vi "testBench-0#-enumTest.vi"() -> ()   [LabVIEW 2015]
doc: "该模板用于创建生产者／消费者模式的应用程序，以事件驱动的方式，生成队列中的项。如需通过响应事件实现代码的异步执行，同时不影响用户界面的响应速度，可考虑用该模式替代用户界面事件处理器模式。"
panel:
  out "ms":cluster{u32, u32, u32, u32, u32}
  out "算法耗时ms":u32
  out "路径":path
  out "出料信息":enum16{"未检", "废品", "尺寸", "外观", "良品"}(ring)=enum."良品"
  in  "各镜槽向配置修正量":dbl[](array[numeric])=[0.0, 0.0, 0.0, 0.0, 0.0, 0.0, 0.0, 0.0, 0.0, 0.0]
  out "#0判定结果显示":T1={"槽宽最大值"=100.0, "槽宽OK"=FALSE, "铜碎OK"=FALSE, "镀锡OK"=FALSE, "白条OK"=TRUE, "头缺OK"=TRUE, "镜角数值"=0}
  in  "检测控制参数 2":cluster{"槽数":i32, "槽宽上限":dbl, "白条面积上限":dbl}={"槽数"=3, "槽宽上限"=12.0, "白条面积上限"=50.0}
  in  "自动运行":bool
  in  "Quit":bool
  out "完成":bool=TRUE
  in  "文件路径（使用对话框）":path=path "D:/IMGFILES/180404/刀纹/cam5/NG"
  out "Display Image":T2(plugin-control)
  in  "输入簇":errorcluster
  in  "Enqueue Element":bool caption="元素入队列"
  in  "stop":bool caption="停止"
  # "可将错误或警告信息Overlay至图像显示，便于检视"
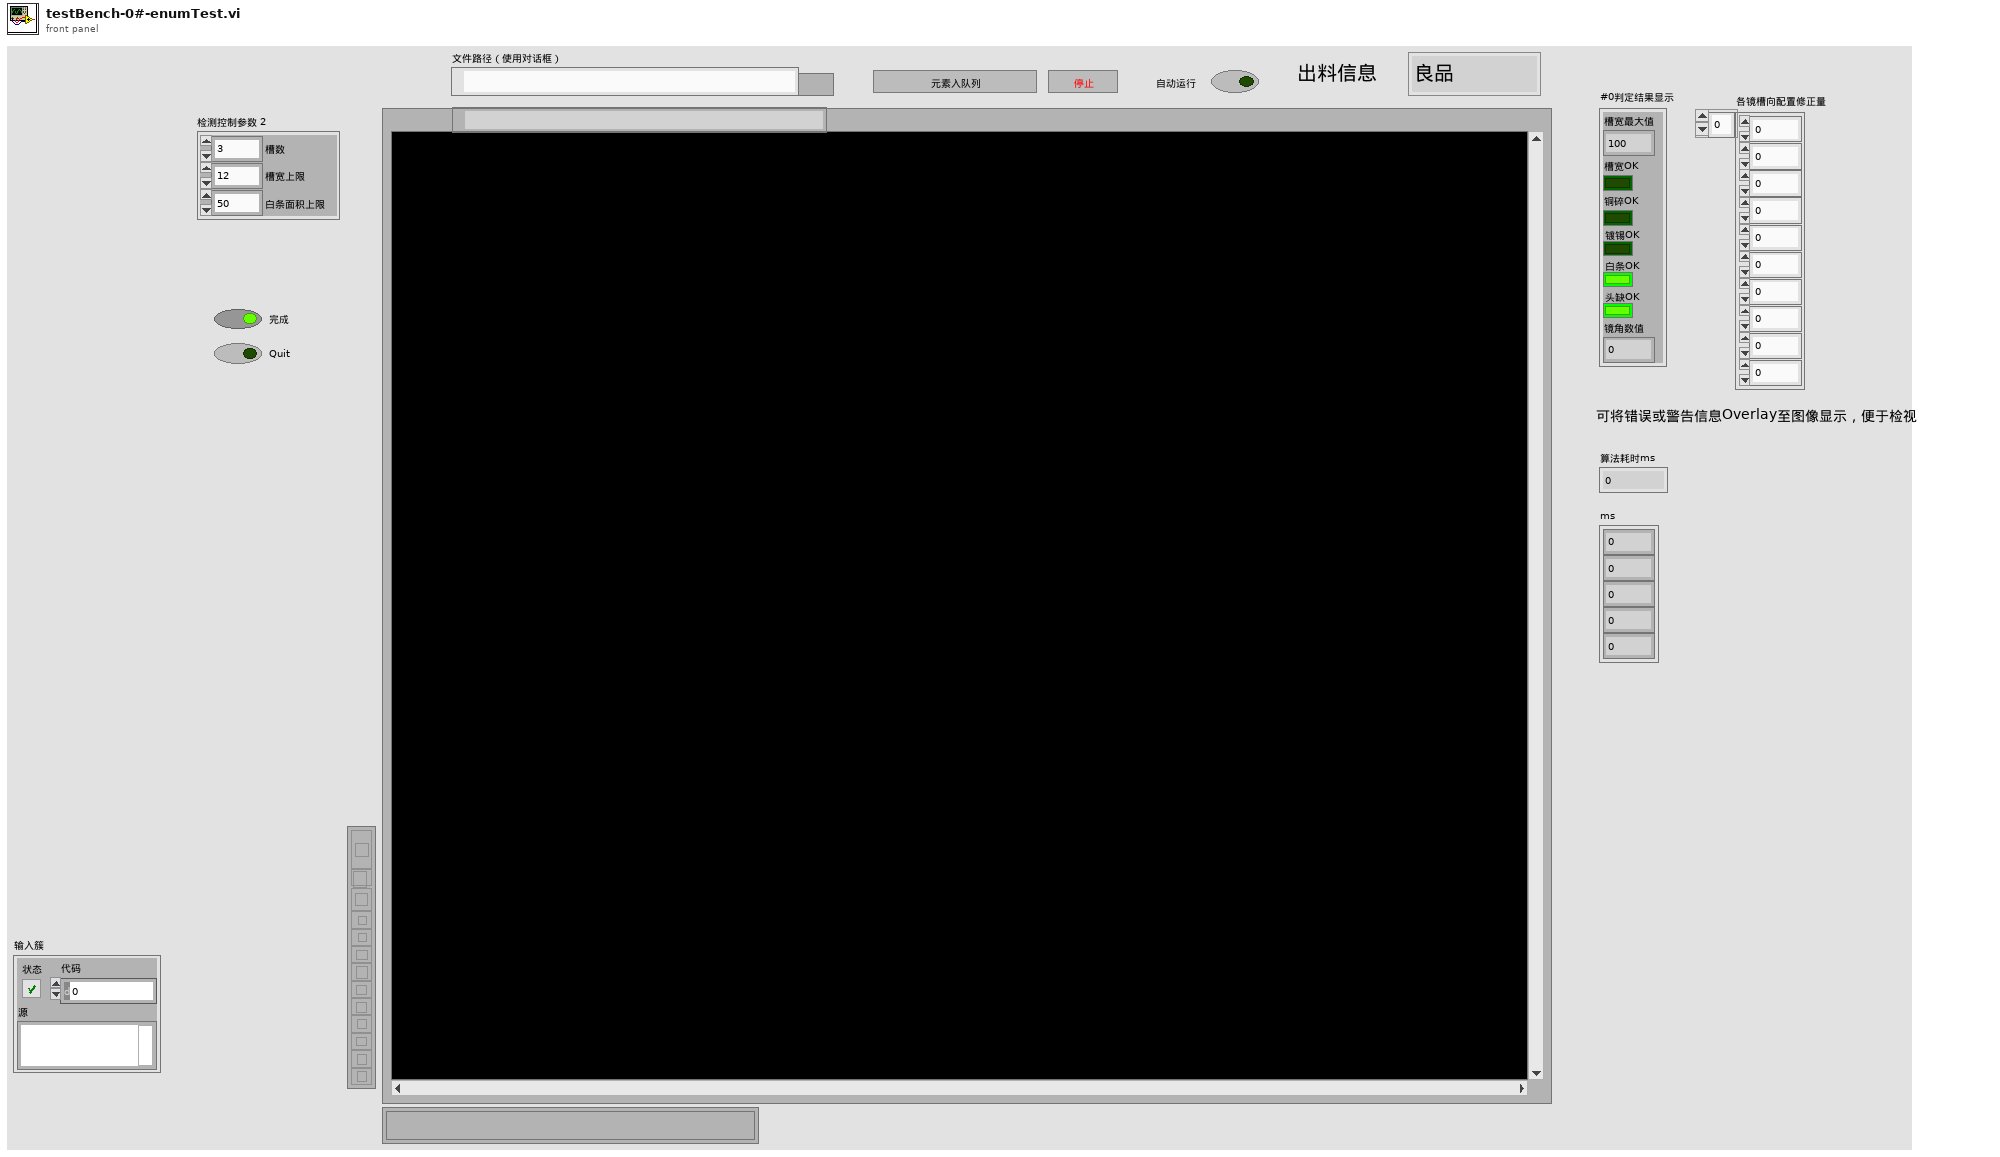
[diagram p1: front panel]
types:
  T1 = cluster{"槽宽最大值":sgl, "槽宽OK":bool, "铜碎OK":bool, "镀锡OK":bool, "白条OK":bool, "头缺OK":bool, "镜角数值":u32}
  T2 = typedef "IMAQ Image.ctl" = refnum<image>
  T3 = typedef "Image Type" = u32
  T4 = cluster{"New Image":T2, "New Image":T2, "New Image":T2, "New Image":T2, "New Image":T2, "New Image":T2, "New Image":T2, "New Image":T2, "New Image":T2, "New Image":T2, "New Image":T2, "New Image":T2, "New Image":T2, "New Image":T2, "New Image":T2, "New Image 2":T2, "New Image 3":T2, "New Image 4":T2}
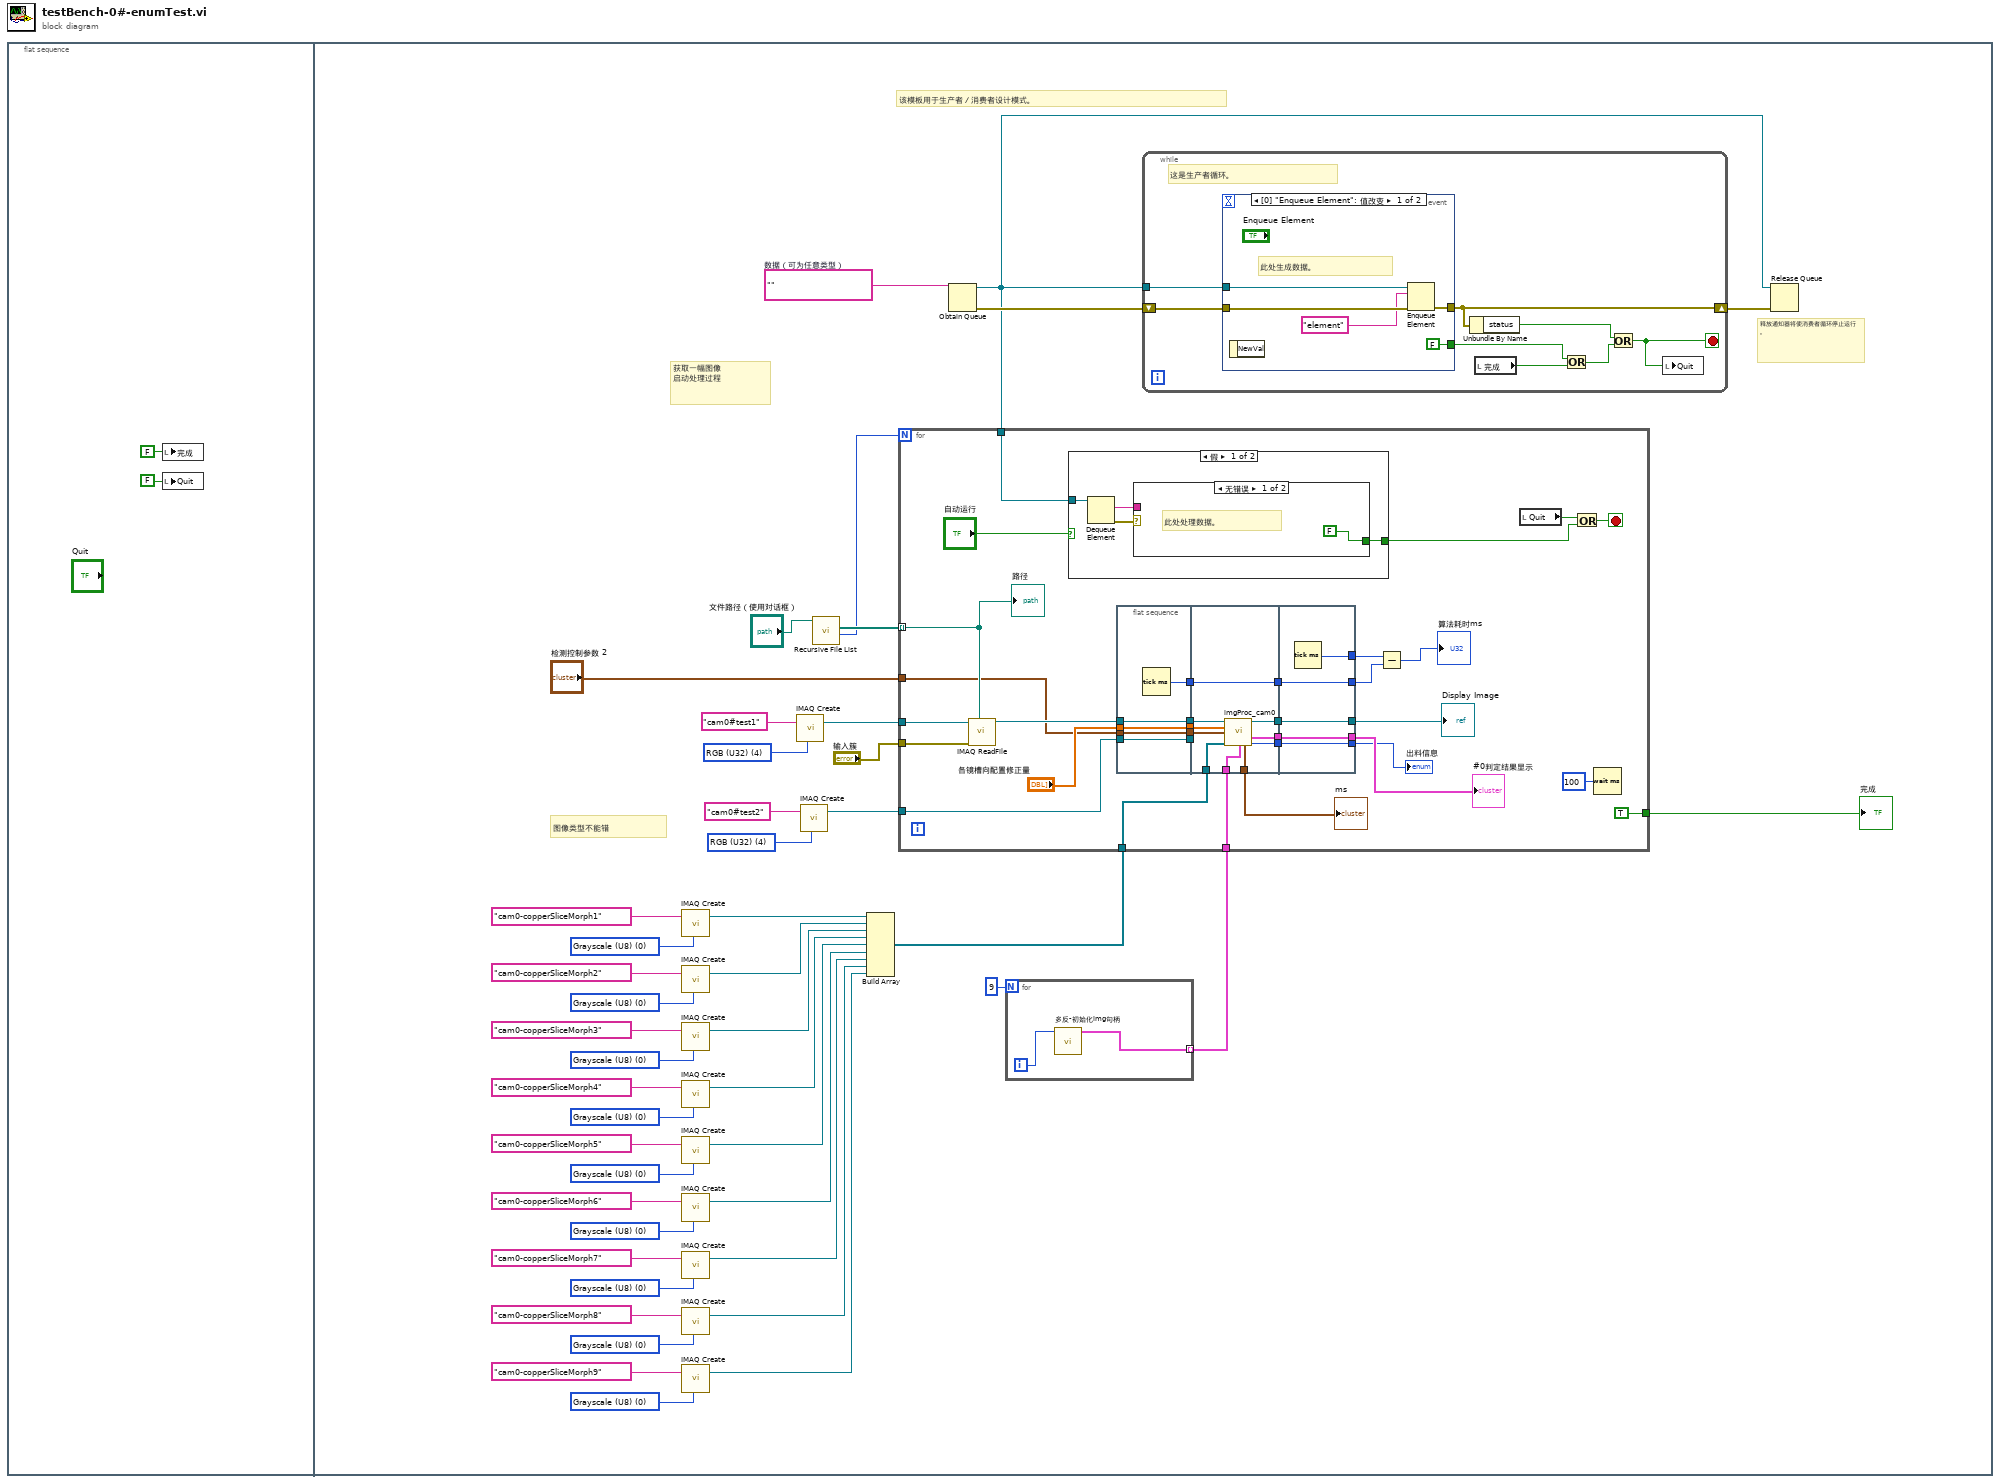
[diagram p0: block diagram]
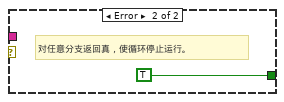
[diagram p2: hidden frame]
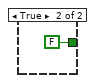
[diagram p3: hidden frame]
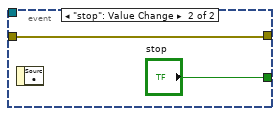
[diagram p4: hidden frame]
diagram:
  n1 = flat-sequence {
    frame #0 {
      n2 = local write "完成"(FALSE ("完成")) -> ()
      n3 = local write "Quit"(FALSE ("完成")) -> ()
    }
    frame #1 {
      w9 = T3 0 items=["Grayscale (U8)", "Grayscale (I16)", "Grayscale (SGL)", "Complex (CSG)", "RGB (U32)", "HSL (U32)", "RGB (U64)", "Grayscale (U16)"] ("Image Type")
      w12 = T3 0 items=["Grayscale (U8)", "Grayscale (I16)", "Grayscale (SGL)", "Complex (CSG)", "RGB (U32)", "HSL (U32)", "RGB (U64)", "Grayscale (U16)"] ("Image Type")
      w13 = T3 0 items=["Grayscale (U8)", "Grayscale (I16)", "Grayscale (SGL)", "Complex (CSG)", "RGB (U32)", "HSL (U32)", "RGB (U64)", "Grayscale (U16)"] ("Image Type")
      w26 = T3 0 items=["Grayscale (U8)", "Grayscale (I16)", "Grayscale (SGL)", "Complex (CSG)", "RGB (U32)", "HSL (U32)", "RGB (U64)", "Grayscale (U16)"] ("Image Type")
      w23 = T3 0 items=["Grayscale (U8)", "Grayscale (I16)", "Grayscale (SGL)", "Complex (CSG)", "RGB (U32)", "HSL (U32)", "RGB (U64)", "Grayscale (U16)"] ("Image Type")
      w22 = T3 0 items=["Grayscale (U8)", "Grayscale (I16)", "Grayscale (SGL)", "Complex (CSG)", "RGB (U32)", "HSL (U32)", "RGB (U64)", "Grayscale (U16)"] ("Image Type")
      w27 = T3 0 items=["Grayscale (U8)", "Grayscale (I16)", "Grayscale (SGL)", "Complex (CSG)", "RGB (U32)", "HSL (U32)", "RGB (U64)", "Grayscale (U16)"] ("Image Type")
      w30 = T3 0 items=["Grayscale (U8)", "Grayscale (I16)", "Grayscale (SGL)", "Complex (CSG)", "RGB (U32)", "HSL (U32)", "RGB (U64)", "Grayscale (U16)"] ("Image Type")
      w31 = T3 0 items=["Grayscale (U8)", "Grayscale (I16)", "Grayscale (SGL)", "Complex (CSG)", "RGB (U32)", "HSL (U32)", "RGB (U64)", "Grayscale (U16)"] ("Image Type")
      w35 = T3 4 items=["Grayscale (U8)", "Grayscale (I16)", "Grayscale (SGL)", "Complex (CSG)", "RGB (U32)", "HSL (U32)", "RGB (U64)", "Grayscale (U16)"] ("Image Type")
      w45 = T3 4 items=["Grayscale (U8)", "Grayscale (I16)", "Grayscale (SGL)", "Complex (CSG)", "RGB (U32)", "HSL (U32)", "RGB (U64)", "Grayscale (U16)"] ("Image Type")
      w46 = ""  # 数据（可为任意类型）
      # "获取一幅图像\n启动处理过程"
      # "图像类型不能错"
      # "释放通知器将使消费者循环停止运行。"
      # "该模板用于生产者／消费者设计模式。"
      n4 = call "IMAQ Create"("Image Name"="cam0-copperSliceMorph1", "Image Type"=w31) -> ("New Image"=w20:T2)  [unwired: 3 in, 1 out]
      n5 = call "IMAQ Create"("Image Name"="cam0-copperSliceMorph2", "Image Type"=w30) -> ("New Image"=w19:T2)  [unwired: 3 in, 1 out]
      n6 = call "IMAQ Create"("Image Name"="cam0-copperSliceMorph3", "Image Type"=w27) -> ("New Image"=w18:T2)  [unwired: 3 in, 1 out]
      n7 = call "IMAQ Create"("Image Name"="cam0-copperSliceMorph4", "Image Type"=w22) -> ("New Image"=w17:T2)  [unwired: 3 in, 1 out]
      n8 = call "IMAQ Create"("Image Name"="cam0-copperSliceMorph5", "Image Type"=w23) -> ("New Image"=w16:T2)  [unwired: 3 in, 1 out]
      n9 = call "IMAQ Create"("Image Name"="cam0-copperSliceMorph6", "Image Type"=w26) -> ("New Image"=w15:T2)  [unwired: 3 in, 1 out]
      n10 = call "IMAQ Create"("Image Name"="cam0-copperSliceMorph7", "Image Type"=w13) -> ("New Image"=w8:T2)  [unwired: 3 in, 1 out]
      n11 = call "IMAQ Create"("Image Name"="cam0-copperSliceMorph8", "Image Type"=w12) -> ("New Image"=w7:T2)  [unwired: 3 in, 1 out]
      n12 = call "IMAQ Create"("Image Name"="cam0-copperSliceMorph9", "Image Type"=w9) -> ("New Image"=w6:T2)  [unwired: 3 in, 1 out]
      n13 = call "IMAQ Create"("Image Name"="cam0#test1", "Image Type"=w45) -> ("New Image"=w39:T2)  [unwired: 3 in, 1 out]
      n14 = call "IMAQ Create"("Image Name"="cam0#test2", "Image Type"=w35) -> ("New Image"=w34:T2)  [unwired: 3 in, 1 out]
      n15 = call <vilib>:"Recursive File List.vi"("Folder Path"="文件路径（使用对话框）") -> ("Number of Files"=w40:i32, "All Files in Dir"=w43:path[])  [unwired: 6 in, 3 out]
      n16 = Build Array(w20, w19, w18, w17, w16, w15, w8, w7, w6) -> (w5:T2[])
      n17 = Obtain Queue(element data type=w46) -> (queue out=w38:refnum<queue>, error out=w48:errorcluster)  [unwired: 4 in, 1 out]
      n18 = for {
        N: 9 -> [_]
        tunnel: [w49] -> w4 mode=indexing
        i -> [w50]
        n19 = call "多反-初始化img句柄.vi"("idx"=w50) -> ("imgDFs"=w49:T4)  [unwired: 10 in]
      }
      n20 = for {
        N: w40 -> [_]
        tunnel: w39 -> [w82]
        tunnel: w43 -> [w80] mode=indexing
        tunnel: "输入簇" -> [w81]
        tunnel: w38 -> [w78]
        tunnel: [TRUE] -> w37
        tunnel: w34 -> [w71]
        tunnel: "检测控制参数 2" -> [w67]
        tunnel: w5 -> [w52]
        tunnel: w4 -> [w51]
        stop <- w74 stop-if-true
        n21 = call "IMAQ ReadFile"("File Path"=w80, "error in (no error)"=w81, "Image"=w82) -> ("Image Out"=w72:T2)  [unwired: 4 in, 4 out]
        n22 = case shown="假" "自动运行" {
          tunnel: w78 -> [w106 _]
          tunnel: [w105 FALSE] -> w75
          frame False {
            n23 = Dequeue Element(queue=w106) -> (element=w104:string, error out=w103:errorcluster)  [unwired: 2 in, 2 out]
            n24 = case shown="无错误" w103 {
              tunnel: w104 -> [_ _]
              tunnel: [FALSE TRUE] -> w105
              frame No Error {
                # "此处处理数据。"
              }
              frame Error {
                # "对任意分支返回真，使循环停止运行。"
              }
            }
          }
          frame True {
          }
        }
        n25 = flat-sequence {
          tunnel: w67 -> [w84]
          tunnel: "各镜槽向配置修正量" -> [w85]
          tunnel: w71 -> [w86]
          tunnel: w72 -> [w87]
          tunnel: [w87] -> w65
          tunnel: [w86] -> w64
          tunnel: [w85] -> w63
          tunnel: [w84] -> w62
          tunnel: [w83] -> w57
          tunnel: w65 -> [w96]
          tunnel: w64 -> [_]
          tunnel: w63 -> [w94]
          tunnel: w62 -> [w93]
          tunnel: [w97] -> w61
          tunnel: [w95] -> w60
          tunnel: [w92] -> w59
          tunnel: w57 -> [w91]
          tunnel: [w91] -> w56
          tunnel: [w90] -> w53
          tunnel: w52 -> [w89]
          tunnel: w51 -> [w88]
          tunnel: [w100] -> w66
          tunnel: [w101] -> w69
          tunnel: [w102] -> w73
          tunnel: w61 -> [w102]
          tunnel: w60 -> [w101]
          tunnel: w59 -> [w100]
          tunnel: [w99] -> w58
          tunnel: w56 -> [w98]
          tunnel: [w98] -> w55
          frame #0 {
            n26 = Tick Count (ms)() -> (millisecond timer value=w83:u32)
          }
          frame #1 {
            n27 = call "imgProc_cam0.vi"("Image In"=w96, "各镜产品轴向角度修正量"=w94, "检测控制参数"=w93, "imgDFtmp"=w89, "ImgTmps"=w88) -> ("Image Out"=w97:T2, "#0判定结果显示"=w95:T1, "ms"=w90:cluster{u32, u32, u32, u32, u32}, "出料信息"=w92:enum16{"未检", "废品", "尺寸", "外观", "良品"})  [unwired: 7 in]
          }
          frame #2 {
            n28 = Tick Count (ms)() -> (millisecond timer value=w99:u32)
          }
        }
        n29 = Subtract(x=w58, y=w55) -> (x-y=→"算法耗时ms":u32)
        n30 = local read "Quit"() -> (w76:bool)
        n31 = Or(x=w76, y=w75) -> (x .or. y?=w74:bool)
        n32 = Wait (ms)(milliseconds to wait=u32 100 ("等待时间（毫秒）")) -> ()  [unwired: 1 out]
        "Display Image" <- w73
        "路径" <- w80
        "#0判定结果显示" <- w69
        "出料信息" <- w66
        "ms" <- w53
      }
      "完成" <- w37
      n33 = while {
        shift-right: [w115] -> w47
        shift-left: w48 -> [w116]
        tunnel: w38 -> [w117]
        stop <- w110 stop-if-true
        # "这是生产者循环。"
        n34 = event shown="[0] \"Enqueue Element\": 值改变" {
          selector: _ -> [_ _]
          dyn-events: _ -> [_ _]
          timeout: _ -> [_ _]
          tunnel: w117 -> [w122 _]
          tunnel: w116 -> [w121 w123]
          tunnel: [w120 w123] -> w115
          tunnel: [FALSE ("stop") "stop"] -> w112
          event "Enqueue Element": Value Change {
            # "此处生成数据。"
            n35 = event-data() -> ()  [unwired: 1 in, 1 out]
            n36 = Enqueue Element(queue=w122, element="element", error in (no error)=w121) -> (error out=w120:errorcluster)  [unwired: 1 in, 2 out]
          }
          event "stop": Value Change {
            n37 = event-data() -> ()  [unwired: 1 in, 1 out]
          }
        }
        n38 = Unbundle By Name(w115) -> ("status"=w114:bool)
        n39 = local read "完成"() -> (w113:bool)
        n40 = Or(x=w112, y=w113) -> (x .or. y?=w111:bool)
        n41 = Or(x=w114, y=w111) -> (x .or. y?=w110:bool)
        n42 = local write "Quit"(w110) -> ()
      }
      n43 = Release Queue(queue=w38, error in (no error)=w47) -> ()  [unwired: 1 in, 3 out]
    }
  }
